vi "测量数据插入数据库.vi"(8 "error in (no error)":errorcluster, 11 "data":T1={"时间"=timestamp(0 s since 1904-01-01), "测量模式"="", "数据类型"="", "检测值"=0.0, "单位"="", "数据标识"="N", "因子编码"="w01019", "标样参考值"=0.0, "ORP-A"=0.0, "ORP-B"=0.0, "ORP-K"=0.0, "COD滴定值"=0.0, "高锰酸钾滴定数"=0.0, "温度"=0.0}) -> (0 "error out":errorcluster)   [LabVIEW 2016, in "一代CodMn.lvlib"]
uses:
  <vilib>/Utility/sysdir.llb/System Directory Type.ctl
  <vilib>/addons/database/Connection.llb/DB Tools Open Connec (String).vi
  <vilib>/addons/database/NI_Database_API.lvlib
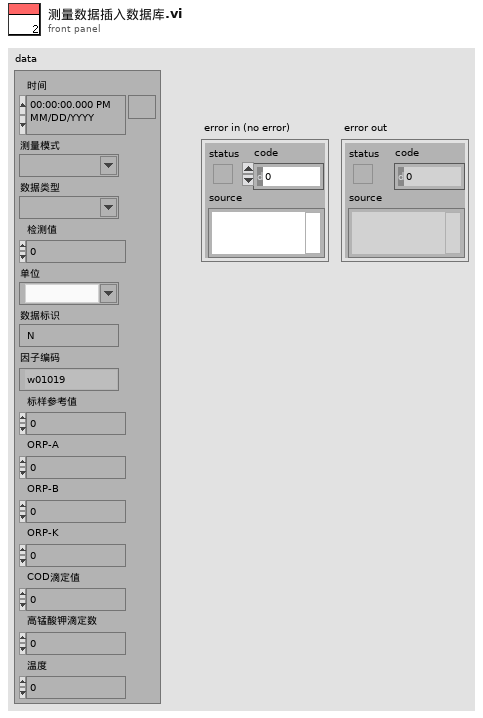
[diagram p1: front panel]
types:
  T1 = cluster{"时间":timestamp, "测量模式":string, "数据类型":string, "检测值":sgl, "单位":string, "数据标识":string, "因子编码":string, "标样参考值":sgl, "ORP-A":sgl, "ORP-B":sgl, "ORP-K":sgl, "COD滴定值":sgl, "高锰酸钾滴定数":sgl, "温度":sgl}
  T2 = typedef "System Directory Type.ctl" = i32
  T3 = typedef "NI_Database_API.lvlib/Conn ObjectReference.ctl" = refnum<k1>
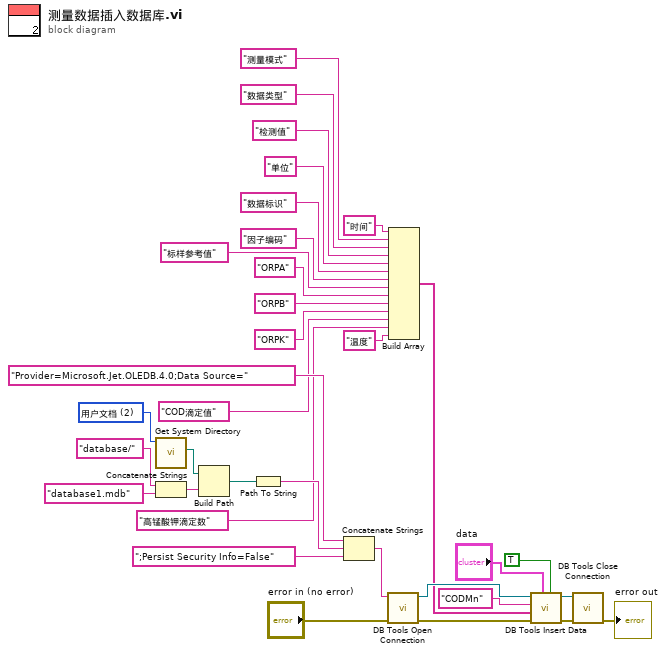
[diagram p0: block diagram]
diagram:
  w31 = T2 2 items=["用户目录"=0, "用户桌面"=1, "用户文档"=2, "用户应用程序数据"=3, "用户设置"=4, "用户临时目录"=5, "公共文档"=6, "公共应用程序数据"=7, "公共设置"=8, "公共缓存"=13, "系统核心库"=9, "系统安装库"=10, "应用程序文件"=11, "启动盘根目录"=12] ("system directory type")
  n1 = call <vilib>:"Get System Directory.vi"("system directory type"=w31) -> ("system directory"=w29:path)  [unwired: 10 in]
  n2 = Concatenate Strings("database/" ("condition"), "database1.mdb" ("字符串")) -> (w22:string)
  n3 = Build Path(base path=w29, name or relative path=w22) -> (appended path=w28:path)
  n4 = Path To String(path=w28) -> (string=w27:string)
  n5 = Concatenate Strings("Provider=Microsoft.Jet.OLEDB.4.0;Data Source=" ("condition"), w27, ";Persist Security Info=False" ("condition")) -> (w25:string)
  n6 = call-poly <vilib>:"DB Tools Open Connection.vi"("error in (no error)"="error in (no error)", "connection information"=w25) -> ("error out"=w23:errorcluster, "connection reference"=w24:T3)  [unwired: 6 in]
  n7 = Build Array("时间", "测量模式", "数据类型", "检测值", "单位", "数据标识", "因子编码", "标样参考值", "ORPA", "ORPB", "ORPK", "COD滴定值", "高锰酸钾滴定数", "温度") -> (w3:string[])
  n8 = call <vilib>:"DB Tools Insert Data.vi"("create table? (F)"=TRUE, "data"="data", "error in (no error)"=w23, "columns"=w3, "table"="CODMn", "connection reference"=w24) -> ("error out"=w33:errorcluster, "connection reference out"=w34:T3)  [unwired: 4 in]
  n9 = call <vilib>:"DB Tools Close Connection.vi"("error in (no error)"=w33, "connection reference"=w34) -> ("error out"=→"error out":errorcluster)  [unwired: 5 in]
